vi "LVIS_CalcMeasResult.vi"(8 "Error In":errorcluster, 10 "Log Step?":bool, 11 "Value":string) -> (0 "Error out":errorcluster, 3 "MeasInfo":T1)   [LabVIEW 2015]
doc: "Determines the measurement status based on the value, type, LL, LL Comp, HL and HL Comp."
uses:
  Globals/LVIS_IsGlobal.vi
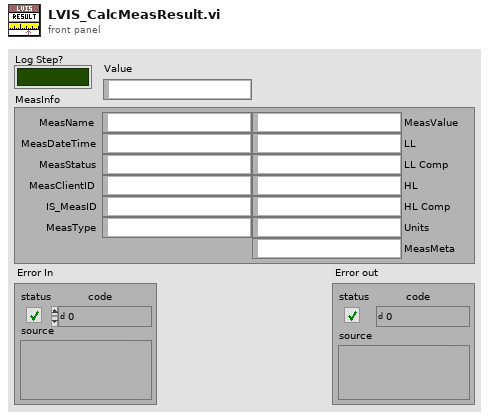
[diagram p1: front panel]
types:
  T1 = cluster{"MeasName":string, "MeasDateTime":string, "MeasStatus":string, "MeasClientID":string, "IS_MeasID":string, "MeasType":string, "MeasValue":string, "LL":string, "LL Comp":string, "HL":string, "HL Comp":string, "Units":string, "MeasMeta":string}
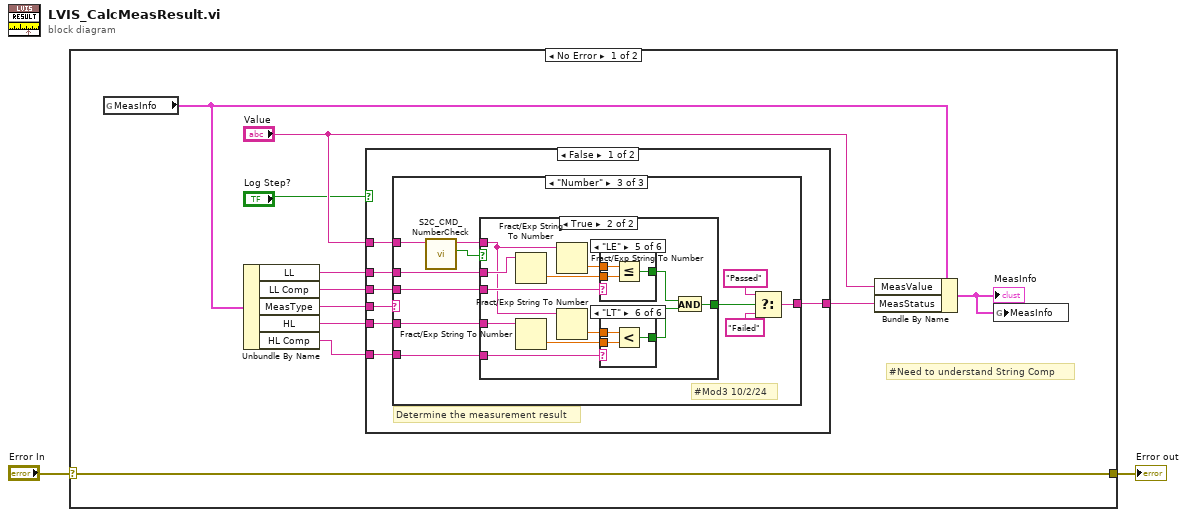
[diagram p0: block diagram]
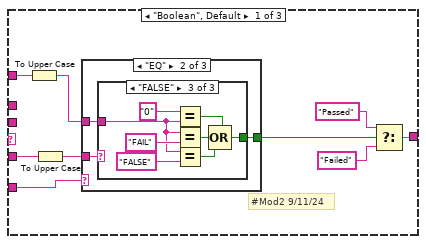
[diagram p2: hidden frame]
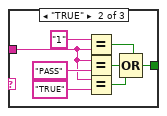
[diagram p5: hidden frame]
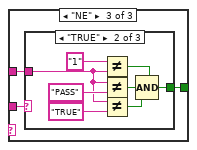
[diagram p6: hidden frame]
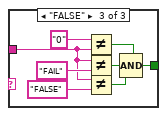
[diagram p8: hidden frame]
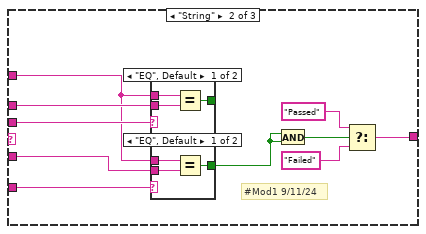
[diagram p9: hidden frame]
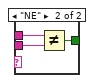
[diagram p10: hidden frame]
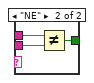
[diagram p11: hidden frame]
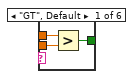
[diagram p13: hidden frame]
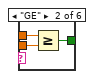
[diagram p14: hidden frame]
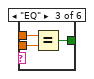
[diagram p15: hidden frame]
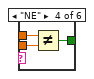
[diagram p16: hidden frame]
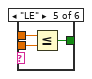
[diagram p17: hidden frame]
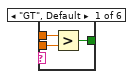
[diagram p18: hidden frame]
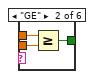
[diagram p19: hidden frame]
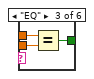
[diagram p20: hidden frame]
diagram:
  n1 = case shown="No Error" "Error In" {
    selector: "Error In" -> [w13 w150]
    tunnel: [w13 w150] -> w1
    frame No Error {
      # "#Need to understand String Comp"
      n2 = global read "LVIS_IsGlobal.vi" "MeasInfo"() -> (w9:T1)
      n3 = Unbundle By Name(w9) -> ("LL"=w11:string, "LL Comp"=w12:string, "MeasType"=w10:string, "HL"=w7:string, "HL Comp"=w8:string)
      n4 = case shown="False" "Log Step?" {
        tunnel: w12 -> [w20 _]
        tunnel: w11 -> [w19 _]
        tunnel: w10 -> [w18 _]
        tunnel: w8 -> [w17 _]
        tunnel: w7 -> [w16 _]
        tunnel: "Value" -> [w15 _]
        tunnel: [w14 "Logged" ("y")] -> w5
        frame False {
          # "Determine the measurement result"
          n5 = case shown="\"Number\"" w18 {
            tunnel: w20 -> [_ w77 w100]
            tunnel: w19 -> [_ w76 w99]
            tunnel: w15 -> [w29 w73 w92]
            tunnel: w17 -> [w21 w71 w98]
            tunnel: w16 -> [w23 w72 w97]
            tunnel: [w25 w70 w93] -> w14
            frame "Boolean", Default {
              # "#Mod2 9/11/24"
              n6 = To Upper Case(1:w29) -> (0:w24:string)
              n7 = To Upper Case(1:w23) -> (0:w22:string)
              n8 = case shown="\"EQ\"" w21 {
                tunnel: [_ w32 w51] -> w26
                tunnel: w24 -> [_ w31 w50]
                tunnel: w22 -> [_ w30 w49]
                frame "Other", Default {
                }
                frame "EQ" {
                  n9 = case shown="\"FALSE\"" w30 {
                    tunnel: [_ w37 w45] -> w32
                    tunnel: w31 -> [_ w34 w42]
                    frame "Other", Default {
                    }
                    frame "TRUE" {
                      n10 = Equal?(x="1", y=w34) -> (x = y?=w40:bool)
                      n11 = Equal?(x=w34, y="PASS") -> (x = y?=w39:bool)
                      n12 = Equal?(x=w34, y="TRUE") -> (x = y?=w33:bool)
                      n13 = Compound Arithmetic op=OR(w40, w39, w33) -> (w37:bool)
                    }
                    frame "FALSE" {
                      n14 = Equal?(x="0", y=w42) -> (x = y?=w48:bool)
                      n15 = Equal?(x=w42, y="FAIL") -> (x = y?=w47:bool)
                      n16 = Equal?(x=w42, y="FALSE") -> (x = y?=w41:bool)
                      n17 = Compound Arithmetic op=OR(w48, w47, w41) -> (w45:bool)
                    }
                  }
                }
                frame "NE" {
                  n18 = case shown="\"TRUE\"" w49 {
                    tunnel: [_ w56 w64] -> w51
                    tunnel: w50 -> [_ w53 w61]
                    frame "Other", Default {
                    }
                    frame "TRUE" {
                      n19 = Not Equal?(x="1", y=w53) -> (x != y?=w59:bool)
                      n20 = Not Equal?(x=w53, y="PASS") -> (x != y?=w58:bool)
                      n21 = Not Equal?(x=w53, y="TRUE") -> (x != y?=w52:bool)
                      n22 = Compound Arithmetic op=AND(w59, w58, w52) -> (w56:bool)
                    }
                    frame "FALSE" {
                      n23 = Not Equal?(x="0", y=w61) -> (x != y?=w67:bool)
                      n24 = Not Equal?(x=w61, y="FAIL") -> (x != y?=w66:bool)
                      n25 = Not Equal?(x=w61, y="FALSE") -> (x != y?=w60:bool)
                      n26 = Compound Arithmetic op=AND(w67, w66, w60) -> (w64:bool)
                    }
                  }
                }
              }
              n27 = Select(t="Passed" ("y"), s=w26, f="Failed" ("y")) -> (s? t:f=w25:string)
            }
            frame "String" {
              # "#Mod1 9/11/24"
              n28 = case shown="\"EQ\", Default" w77 {
                tunnel: w73 -> [w86 w89]
                tunnel: w76 -> [w85 w88]
                tunnel: [w84 w87] -> _
                frame "EQ", Default {
                  n29 = Equal?(x=w86, y=w85) -> (x = y?=w84:bool)
                }
                frame "NE" {
                  n30 = Not Equal?(x=w89, y=w88) -> (x != y?=w87:bool)
                }
              }
              n31 = case shown="\"EQ\", Default" w71 {
                tunnel: w73 -> [w80 w83]
                tunnel: w72 -> [w79 w82]
                tunnel: [w78 w81] -> w68
                frame "EQ", Default {
                  n32 = Equal?(x=w80, y=w79) -> (x = y?=w78:bool)
                }
                frame "NE" {
                  n33 = Not Equal?(x=w83, y=w82) -> (x != y?=w81:bool)
                }
              }
              n34 = And(x=w68, y=w68) -> (x .and. y?=w69:bool)
              n35 = Select(t="Passed" ("y"), s=w69, f="Failed" ("y")) -> (s? t:f=w70:string)
            }
            frame "Number" {
              # "#Mod3 10/2/24"
              n36 = call "S2C_CMD_NumberCheck.vi"("String In"=w92) -> ("Is Number?"=w90:bool, "String Out"=w91:string)  [unwired: 8 in, 1 out]
              n37 = case shown="True" w90 {
                tunnel: w100 -> [_ w112]
                tunnel: w99 -> [_ w110]
                tunnel: w98 -> [_ w106]
                tunnel: w97 -> [_ w105]
                tunnel: w91 -> [_ w104]
                tunnel: [_ w101] -> w94
                frame False {
                }
                frame True {
                  n38 = Fract/Exp String To Number(string=w110) -> (number=w109:dbl)  [unwired: 3 in, 1 out]
                  n39 = Fract/Exp String To Number(string=w105) -> (number=w108:dbl)  [unwired: 3 in, 1 out]
                  n40 = Fract/Exp String To Number(string=w104) -> (number=w111:dbl)  [unwired: 3 in, 1 out]
                  n41 = Fract/Exp String To Number(string=w104) -> (number=w107:dbl)  [unwired: 3 in, 1 out]
                  n42 = case shown="\"LE\"" w112 {
                    tunnel: w111 -> [w133 w136 w139 w142 w145 w148]
                    tunnel: w109 -> [w132 w135 w138 w141 w144 w147]
                    tunnel: [w131 w134 w137 w140 w143 w146] -> w103
                    frame "GT", Default {
                      n43 = Greater?(x=w133, y=w132) -> (0:w131:bool)
                    }
                    frame "GE" {
                      n44 = Greater Or Equal?(x=w136, y=w135) -> (x >= y?=w134:bool)
                    }
                    frame "EQ" {
                      n45 = Equal?(x=w139, y=w138) -> (x = y?=w137:bool)
                    }
                    frame "NE" {
                      n46 = Not Equal?(x=w142, y=w141) -> (x != y?=w140:bool)
                    }
                    frame "LE" {
                      n47 = Less Or Equal?(x=w145, y=w144) -> (x <= y?=w143:bool)
                    }
                    frame "LT" {
                      n48 = Less?(x=w148, y=w147) -> (x < y?=w146:bool)
                    }
                  }
                  n49 = case shown="\"LT\"" w106 {
                    tunnel: w107 -> [w115 w118 w121 w124 w127 w130]
                    tunnel: w108 -> [w114 w117 w120 w123 w126 w129]
                    tunnel: [w113 w116 w119 w122 w125 w128] -> w102
                    frame "GT", Default {
                      n50 = Greater?(x=w115, y=w114) -> (0:w113:bool)
                    }
                    frame "GE" {
                      n51 = Greater Or Equal?(x=w118, y=w117) -> (x >= y?=w116:bool)
                    }
                    frame "EQ" {
                      n52 = Equal?(x=w121, y=w120) -> (x = y?=w119:bool)
                    }
                    frame "NE" {
                      n53 = Not Equal?(x=w124, y=w123) -> (x != y?=w122:bool)
                    }
                    frame "LE" {
                      n54 = Less Or Equal?(x=w127, y=w126) -> (x <= y?=w125:bool)
                    }
                    frame "LT" {
                      n55 = Less?(x=w130, y=w129) -> (x < y?=w128:bool)
                    }
                  }
                  n56 = And(x=w103, y=w102) -> (x .and. y?=w101:bool)
                }
              }
              n57 = Select(t="Passed" ("y"), s=w94, f="Failed" ("y")) -> (s? t:f=w93:string)
            }
          }
        }
        frame True {
          # "No Check, status is Logged"
        }
      }
      n58 = Bundle By Name(cluster=w9, "MeasValue"="Value", "MeasStatus"=w5) -> (w4:T1)
      "MeasInfo" <- w4
      n59 = global write "LVIS_IsGlobal.vi" "MeasInfo"(w4) -> ()
    }
    frame Error {
    }
  }
  "Error out" <- w1
